vi "testGameNewUI.vi"() -> ()   [LabVIEW 2024]
uses:
  state machine variables.ctl
  state machine states.ctl
panel:
  out "Sequence":dbl[](array[numeric])
  in  "Difficulty":dbl(slide) scale=2.0..10.0
  in  "Button 4":bool
  in  "Button3":bool
  in  "Button 2":bool
  in  "Button 1":bool
  in  "Pulse or Play":bool caption="Blank Button"
  in  "Exit":bool caption="Blank Button"
  in  "Round":dbl
  in  "Score":dbl
  in  "stop":bool
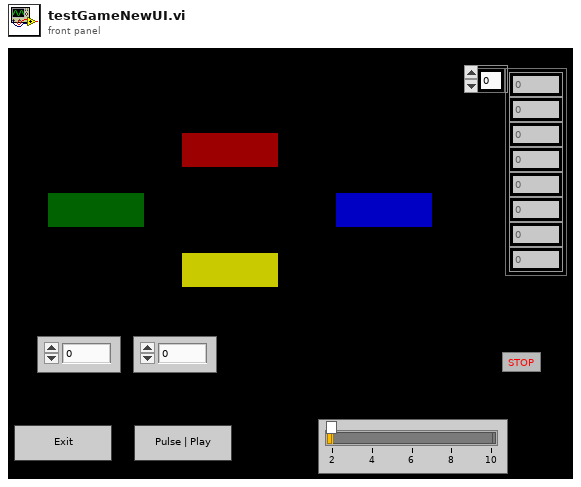
[diagram p1: front panel]
types:
  T1 = typedef "state machine states.ctl" = enum16{"Initialize", "update display", "Show sequence", "User response", "update data", ""}
  T2 = typedef "state machine variables.ctl" = cluster{"Sequence":dbl[], "Score":dbl, "Round":dbl}
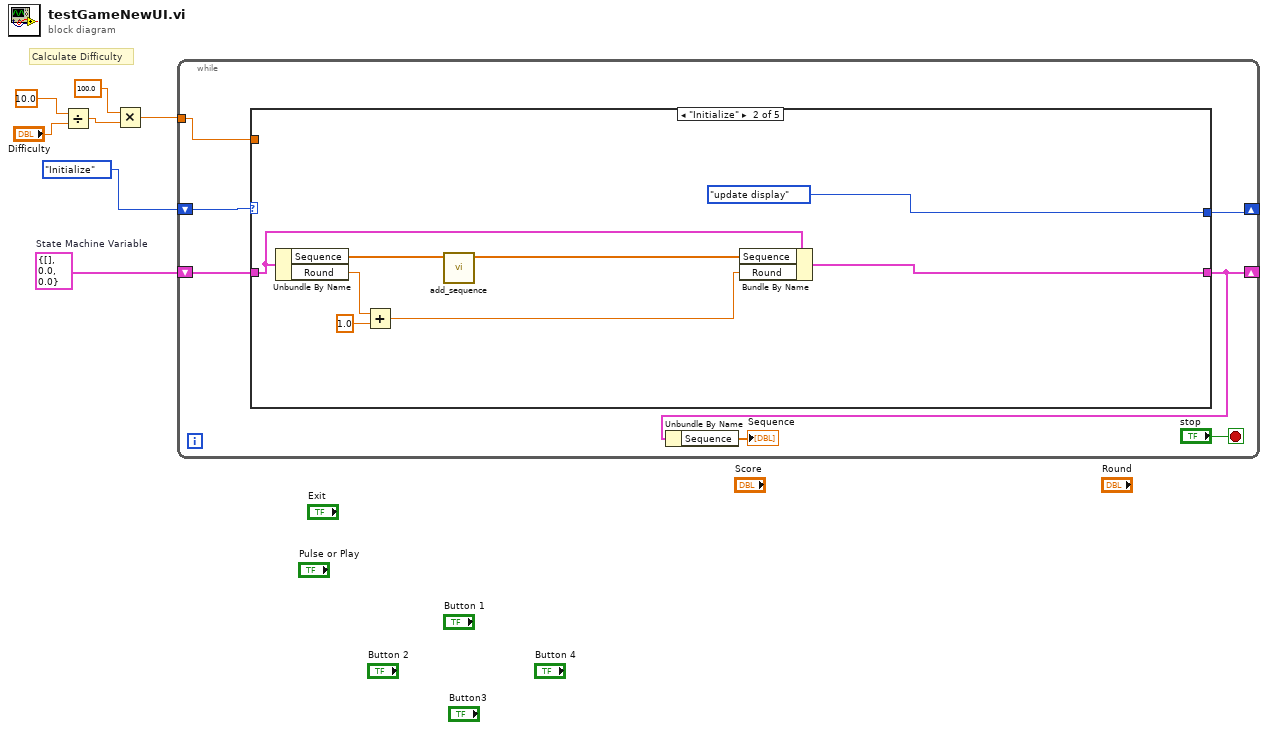
[diagram p0: block diagram]
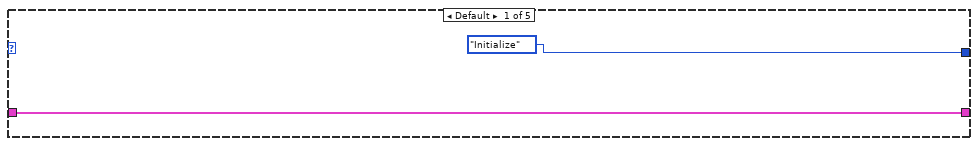
[diagram p2: hidden frame]
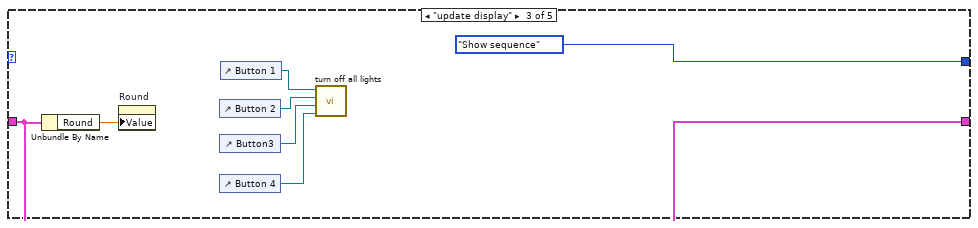
[diagram p3: hidden frame]
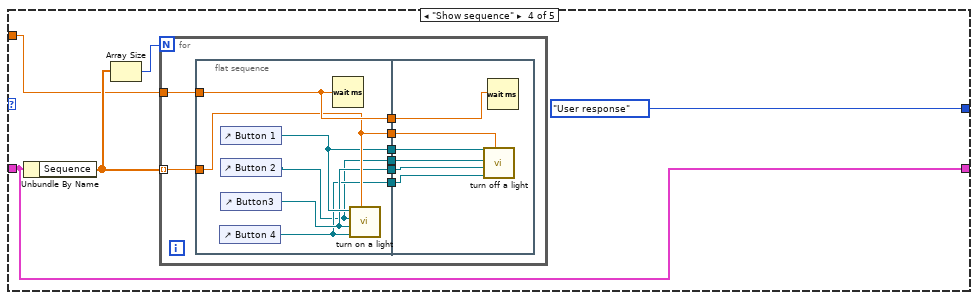
[diagram p4: hidden frame]
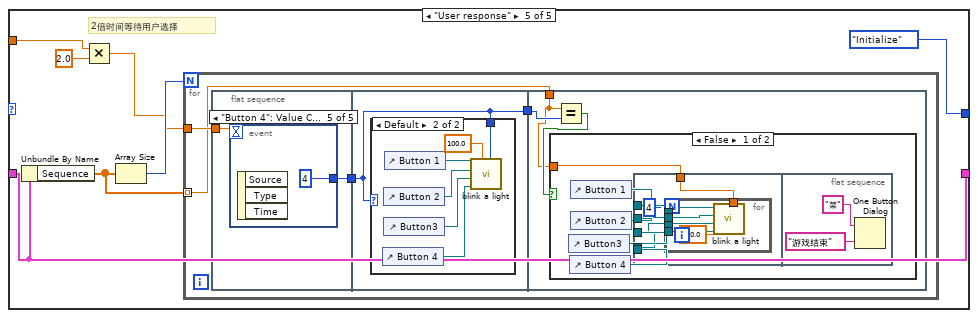
[diagram p5: hidden frame]
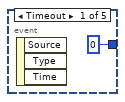
[diagram p6: hidden frame]
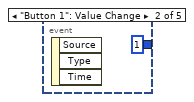
[diagram p7: hidden frame]
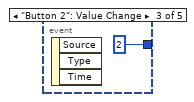
[diagram p8: hidden frame]
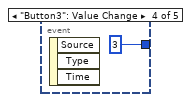
[diagram p9: hidden frame]
diagram:
  w7 = T2 {"Sequence"=[], "Score"=0.0, "Round"=0.0}  # State Machine Variable
  # "Calculate Difficulty"
  n1 = Divide(x=10.0, y="Difficulty") -> (x/y=w3:dbl)
  n2 = Multiply(x=100.0, y=w3) -> (x*y=w2:dbl)
  n3 = while {
    shift-right: [w8] -> _
    shift-left: w7 -> [w14]
    shift-right: [w11] -> _
    shift-left: state_machine_states."Initialize" -> [w12]
    tunnel: w2 -> [w10]
    stop <- "stop" stop-if-true
    n4 = case shown="\"Initialize\"" w12 {
      tunnel: w14 -> [w16 w23 w31 w32 w57]
      tunnel: [w16 w22 w31 w32 w57] -> w8
      tunnel: [state_machine_states."Initialize" ("Enum") state_machine_states."update display" ("Enum") state_machine_states."Show sequence" ("Enum") state_machine_states."User response" ("Enum") state_machine_states."Initialize" ("Enum")] -> w11
      tunnel: w10 -> [_ _ _ w34 w59]
      frame Default {
      }
      frame "Initialize" {
        n5 = Unbundle By Name(w23) -> ("Sequence"=w24:dbl[], "Round"=w19:dbl)
        n6 = Add(x=w19, y=1.0) -> (x+y=w18:dbl)
        n7 = call "add_sequence.vi"("sequence in"=w24) -> ("sequence out"=w21:dbl[])  [unwired: 9 in, 1 out]
        n8 = Bundle By Name(cluster=w23, "Sequence"=w21, "Round"=w18) -> (w22:T2)
      }
      frame "update display" {
        n9 = Unbundle By Name(w31) -> ("Round"=w30:dbl)
        n10 = property on="Round" class="DigNum (strict)"("Value"=w30) -> ()  [unwired: 2 in, 2 out]
        n11 = control-ref of="Button 2"() -> (w27:refnum<vi>)
        n12 = control-ref of="Button3"() -> (w26:refnum<vi>)
        n13 = control-ref of="Button 4"() -> (w25:refnum<vi>)
        n14 = control-ref of="Button 1"() -> (w28:refnum<vi>)
        n15 = call "turn off all lights.vi"("Button 4"=w25, "Button 3"=w26, "Button 2"=w27, "Button 1"=w28) -> ()  [unwired: 7 in, 1 out]
      }
      frame "Show sequence" {
        n16 = Unbundle By Name(w32) -> ("Sequence"=w35:dbl[])
        n17 = Array Size(array=w35) -> (size(s)=w36:i32)
        n18 = for {
          N: w36 -> [_]
          tunnel: w35 -> [w44] mode=indexing
          tunnel: w34 -> [w43]
          n19 = flat-sequence {
            tunnel: w44 -> [w49]
            tunnel: w43 -> [w50]
            tunnel: [w50] -> w42
            tunnel: [w49] -> w41
            tunnel: [w48] -> w40
            tunnel: [w47] -> w39
            tunnel: [w46] -> w38
            tunnel: [w45] -> w37
            tunnel: w42 -> [w56]
            tunnel: w41 -> [w55]
            tunnel: w40 -> [w54]
            tunnel: w39 -> [w53]
            tunnel: w38 -> [w52]
            tunnel: w37 -> [w51]
            frame #0 {
              n20 = control-ref of="Button 4"() -> (w46:refnum<vi>)
              n21 = control-ref of="Button 1"() -> (w48:refnum<vi>)
              n22 = control-ref of="Button 2"() -> (w45:refnum<vi>)
              n23 = control-ref of="Button3"() -> (w47:refnum<vi>)
              n24 = Wait (ms)(milliseconds to wait=w50) -> ()  [unwired: 1 out]
              n25 = call "turn on a light.vi"("Which Button?"=w49, "Button 4"=w46, "Button 3"=w47, "Button 2"=w45, "Button 1"=w48) -> ()  [unwired: 6 in, 1 out]
            }
            frame #1 {
              n26 = call "turn off a light.vi"("Which Button?"=w55, "Button 4"=w52, "Button 3"=w53, "Button 2"=w51, "Button 1"=w54) -> ()  [unwired: 6 in, 1 out]
              n27 = Wait (ms)(milliseconds to wait=w56) -> ()  [unwired: 1 out]
            }
          }
        }
      }
      frame "User response" {
        # "2倍时间等待用户选择"
        n28 = Unbundle By Name(w57) -> ("Sequence"=w61:dbl[])
        n29 = Multiply(x=w59, y=2.0) -> (x*y=w60:dbl)
        n30 = Array Size(array=w61) -> (size(s)=w62:i32)
        n31 = for {
          N: w62 -> [_]
          tunnel: w61 -> [w65] mode=indexing
          tunnel: w60 -> [w67]
          n32 = flat-sequence {
            tunnel: w67 -> [w69]
            tunnel: [w68] -> w66
            tunnel: w66 -> [w75]
            tunnel: [w75] -> w64
            tunnel: w65 -> [w82]
            tunnel: w64 -> [w84]
            frame #0 {
              n33 = event shown="[4] \"Button 4\": Value Change" {
                selector: _ -> [_ _ _ _ _]
                dyn-events: _ -> [_ _ _ _ _]
                timeout: w69 -> [_ _ _ _ _]
                tunnel: [u32 0 1 2 3 u32 4] -> w68
                event Timeout {
                  n34 = event-data() -> ()  [unwired: 1 in, 3 out]
                }
                event "Button 1": Value Change {
                  n35 = event-data() -> ()  [unwired: 1 in, 3 out]
                }
                event "Button 2": Value Change {
                  n36 = event-data() -> ()  [unwired: 1 in, 3 out]
                }
                event "Button3": Value Change {
                  n37 = event-data() -> ()  [unwired: 1 in, 3 out]
                }
                event "Button 4": Value Change {
                  n38 = event-data() -> ()  [unwired: 1 in, 3 out]
                }
              }
            }
            frame #1 {
              n39 = case shown="Default" w75 {
                tunnel: w75 -> [_ w81]
                frame 0 {
                }
                frame Default {
                  n40 = control-ref of="Button 4"() -> (w77:refnum<vi>)
                  n41 = control-ref of="Button 2"() -> (w79:refnum<vi>)
                  n42 = control-ref of="Button3"() -> (w78:refnum<vi>)
                  n43 = control-ref of="Button 1"() -> (w80:refnum<vi>)
                  n44 = call "blink a light.vi"("Whcih Button?"=w81, "Blink Time"=100.0, "Button 4"=w77, "Button 3"=w78, "Button 2"=w79, "Button 1"=w80) -> ()  [unwired: 5 in, 1 out]
                }
              }
            }
            frame #2 {
              n45 = Equal?(x=w82, y=w84) -> (x = y?=w83:bool)
              n46 = case shown="False" w83 {
                tunnel: w82 -> [w89 _]
                frame False {
                  n47 = control-ref of="Button3"() -> (w86:refnum<vi>)
                  n48 = control-ref of="Button 4"() -> (w85:refnum<vi>)
                  n49 = control-ref of="Button 1"() -> (w88:refnum<vi>)
                  n50 = control-ref of="Button 2"() -> (w87:refnum<vi>)
                  n51 = flat-sequence {
                    tunnel: w89 -> [w95]
                    tunnel: w88 -> [w92]
                    tunnel: w87 -> [w91]
                    tunnel: w86 -> [w93]
                    tunnel: [w94] -> _
                    tunnel: w85 -> [w94]
                    frame #0 {
                      n52 = for {
                        N: 4 -> [_]
                        tunnel: w95 -> [w101]
                        tunnel: w94 -> [w100]
                        tunnel: w93 -> [w99]
                        tunnel: w92 -> [w98]
                        tunnel: w91 -> [w97]
                        n53 = call "blink a light.vi"("Whcih Button?"=w101, "Blink Time"=200.0, "Button 4"=w100, "Button 3"=w99, "Button 2"=w97, "Button 1"=w98) -> ()  [unwired: 5 in, 1 out]
                      }
                    }
                    frame #1 {
                      n54 = One Button Dialog(message="菜", button name ("OK")="游戏结束") -> ()  [unwired: 1 out]
                    }
                  }
                }
                frame True {
                }
              }
            }
          }
        }
      }
    }
    n55 = Unbundle By Name(w8) -> ("Sequence"=→"Sequence":dbl[])
  }
